vi "CAN.FG.vi"(7 "Action":T1, 8 "error in (no error)":errorcluster, 10 "Diagnostics Basic Configuration":T2={"Interface"="", "Baud Rate"=0, "Diagnostic Protocol"=enum."GMLAN", "Transport Protocol"=enum."ISO TP - Normal Mode", "Transmit ID"=0, "Receive ID"=0, "Transmit Extension"=0, "Receive Extension"=0, "Receive UUDT ID"=0, "Enable Stream"=TRUE, "VW TP Channel ID"=0, "Fill Frame"=TRUE, "Fill Byte"=255, "Termination"=FALSE, "LIN Cluster"="ADCS_LIN_database", "NAD"=1, "IO Mode"=0, "Max DLC"=8, "FD Baud Rate"=0, "Timeout"=1000, "FD ISO Mode"=0, "DoIP Address"="", "DoIP Source Address"=3584, "DoIP Dynamic Port"=TRUE, "DoIP Version"=2} {"DoIP Version" items=["2010"=1, "2012"=2]; "DoIP Source Address" format="%.0x"; "FD ISO Mode" items=["ISO", "Non ISO", "ISO Legacy"]; "IO Mode" items=["CAN 2.0", "CAN FD", "CAN FD+BRS"]; "Fill Byte" format="%.0x"; "VW TP Channel ID" format="%.0x"; "Receive UUDT ID" format="%.0x"; "Receive Extension" format="%.0x"; "Transmit Extension" format="%.0x"; "Receive ID" format="%.0x"; "Transmit ID" format="%.0x"}, 11 "Device Item Ref in":T6 format="%.0x") -> (0 "error out":errorcluster, 2 "Diagnostics Basic Configuration":T2={"Interface"="", "Baud Rate"=0, "Diagnostic Protocol"=enum."GMLAN", "Transport Protocol"=enum."ISO TP - Normal Mode", "Transmit ID"=0, "Receive ID"=0, "Transmit Extension"=0, "Receive Extension"=0, "Receive UUDT ID"=0, "Enable Stream"=TRUE, "VW TP Channel ID"=0, "Fill Frame"=FALSE, "Fill Byte"=255, "Termination"=FALSE, "LIN Cluster"="ADCS_LIN_database", "NAD"=1, "IO Mode"=0, "Max DLC"=8, "FD Baud Rate"=0, "Timeout"=0, "FD ISO Mode"=0, "DoIP Address"="", "DoIP Source Address"=3584, "DoIP Dynamic Port"=TRUE, "DoIP Version"=2} {"DoIP Version" items=["2010"=1, "2012"=2]; "DoIP Source Address" format="%.0x"; "FD ISO Mode" items=["ISO", "Non ISO", "ISO Legacy"]; "IO Mode" items=["CAN 2.0", "CAN FD", "CAN FD+BRS"]; "Fill Byte" format="%.0x"; "VW TP Channel ID" format="%.0x"; "Receive UUDT ID" format="%.0x"; "Receive Extension" format="%.0x"; "Transmit Extension" format="%.0x"; "Receive ID" format="%.0x"; "Transmit ID" format="%.0x"}, 3 "Device Item Ref out":T6=18446744073709551615 format="%.0x")   [LabVIEW 2019, in "Diagnostics Addon System Explorer.lvlib"]
uses:
  Diagnostics Addon System Explorer.lvlib
  <vilib>/NI VeriStand/Custom Device API/Custom Device Item Ref.ctl
  Addon Shared/Types/CAN.ctl
  Addon Shared/Types/CAN.Interface.ctl
  Addon Shared/Types/Protocol.ctl
  Addon Shared/Types/Transport.ctl
  Types/FG.Action.ctl
  Addon Shared/SubVIs/Constants.vi
  <vilib>/NI VeriStand/Custom Device API/Get Item Property (String).vi
  <vilib>/NI VeriStand/Custom Device API/Get Item Property (Variant).vi
  <vilib>/NI VeriStand/Custom Device API/Get Item Property (U32).vi
  <vilib>/NI VeriStand/Custom Device API/Get Item Property (Boolean).vi
  <vilib>/NI/NI VeriStand Advanced SysDef API/_SubVIs/SysDef.Property.Set.String.vi
  <vilib>/NI/NI VeriStand Advanced SysDef API/_SubVIs/SysDef.Property.Set.Variant.vi
  <vilib>/NI/NI VeriStand Advanced SysDef API/_SubVIs/SysDef.Property.Set.U32.vi
  <vilib>/NI/NI VeriStand Advanced SysDef API/_SubVIs/SysDef.Property.Set.Boolean.vi
  Addon Shared/Diagnostics Addon Shared.lvlib
  <vilib>/NI VeriStand/Custom Device API/Custom Device API.lvlib
  <vilib>/NI/NI VeriStand Advanced SysDef API/SysDef API/Advanced System Definition.lvlib
  <vilib>/NI/NI VeriStand Advanced SysDef API/_SubVIs/SysDef.Property.Set.U16.vi
  <vilib>/NI VeriStand/Custom Device API/Get Item Property (U16).vi
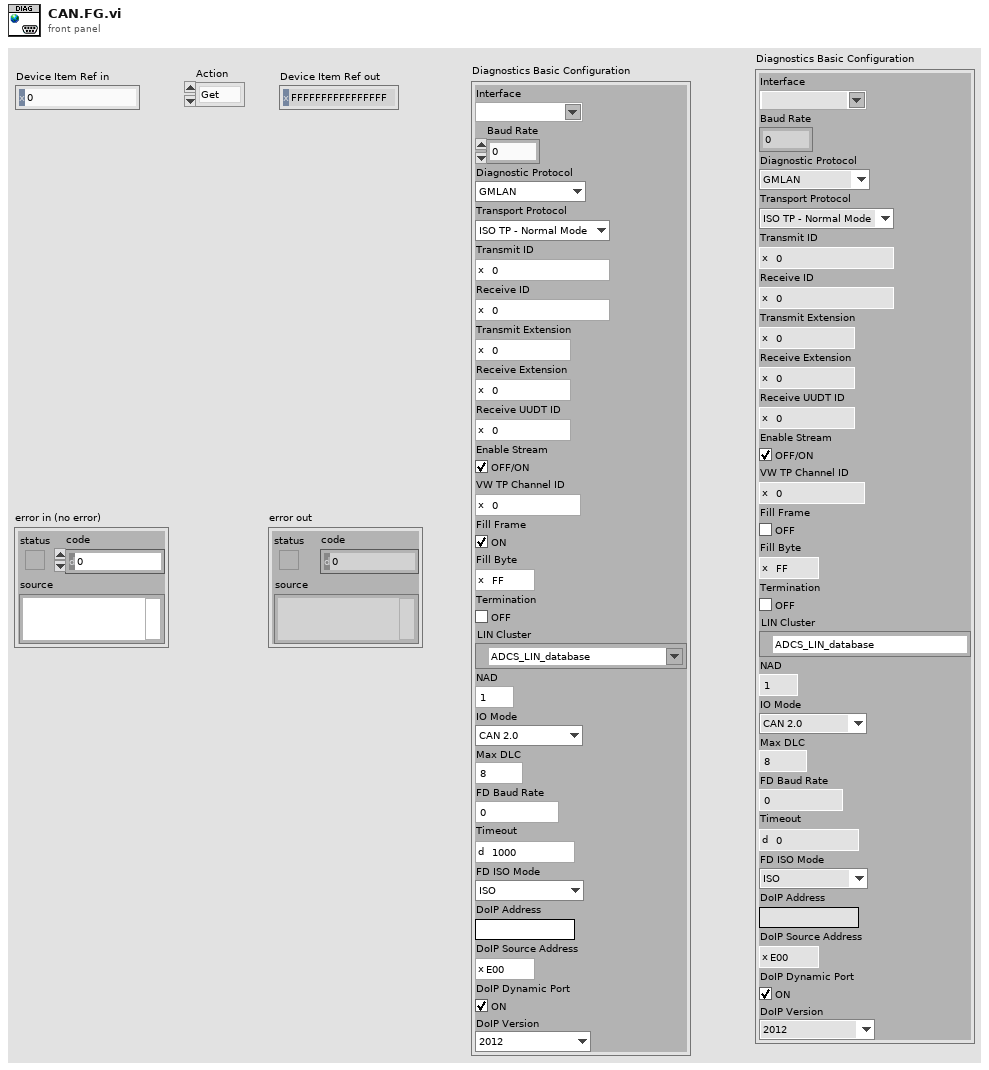
[diagram p1: front panel]
types:
  T1 = typedef "Diagnostics Addon System Explorer.lvlib/FG.Action.ctl" = enum16{"Get", "Set"}
  T2 = typedef "Diagnostics Addon Shared.lvlib/CAN.ctl" = cluster{"Interface":T3, "Baud Rate":u64, "Diagnostic Protocol":T4, "Transport Protocol":T5, "Transmit ID":u32, "Receive ID":u32, "Transmit Extension":u8, "Receive Extension":u8, "Receive UUDT ID":u32, "Enable Stream":bool, "VW TP Channel ID":u32, "Fill Frame":bool, "Fill Byte":u8, "Termination":bool, "LIN Cluster":refnum<k21>, "NAD":u8, "IO Mode":u32, "Max DLC":u16, "FD Baud Rate":u64, "Timeout":u32, "FD ISO Mode":u32, "DoIP Address":string, "DoIP Source Address":u16, "DoIP Dynamic Port":bool, "DoIP Version":u16}
  T3 = typedef "Diagnostics Addon Shared.lvlib/CAN.Interface.ctl" = string
  T4 = typedef "Diagnostics Addon Shared.lvlib/Protocol.ctl" = enum16{"GMLAN", "KWP-2000", "UDS", "User-Defined"}
  T5 = typedef "Diagnostics Addon Shared.lvlib/Transport.ctl" = enum16{"ISO TP - Normal Mode", "ISO TP - Mixed Mode", "VW TP 2.0", "Diagnostics on IP", "ISO TP LIN"}
  T6 = typedef "Custom Device API.lvlib/Custom Device Item Ref.ctl" = u64
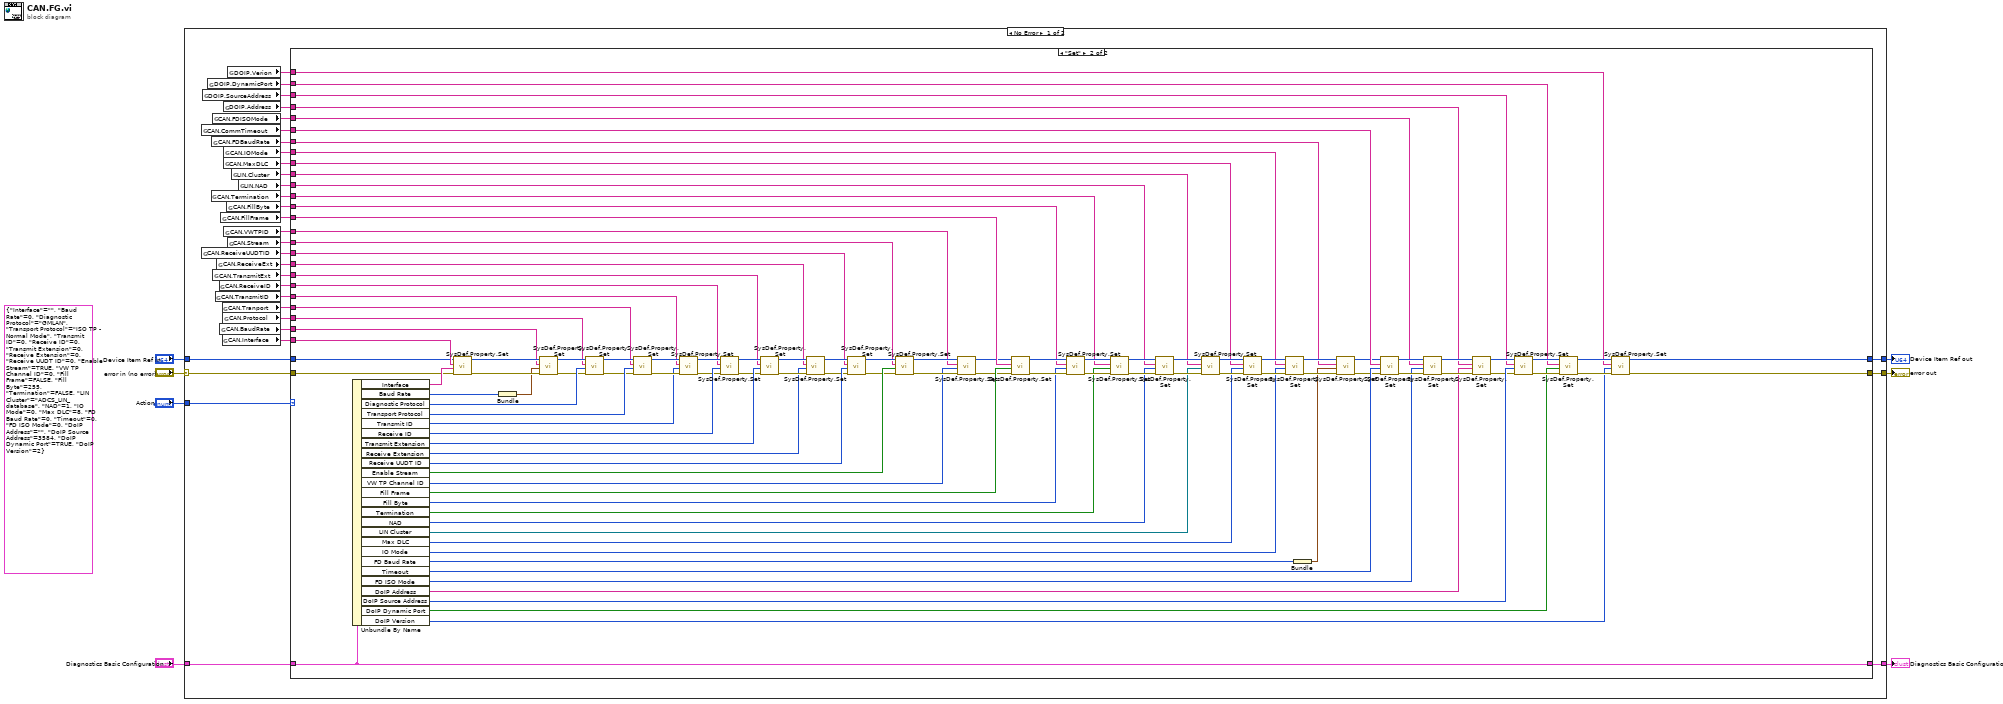
[diagram p0: block diagram]
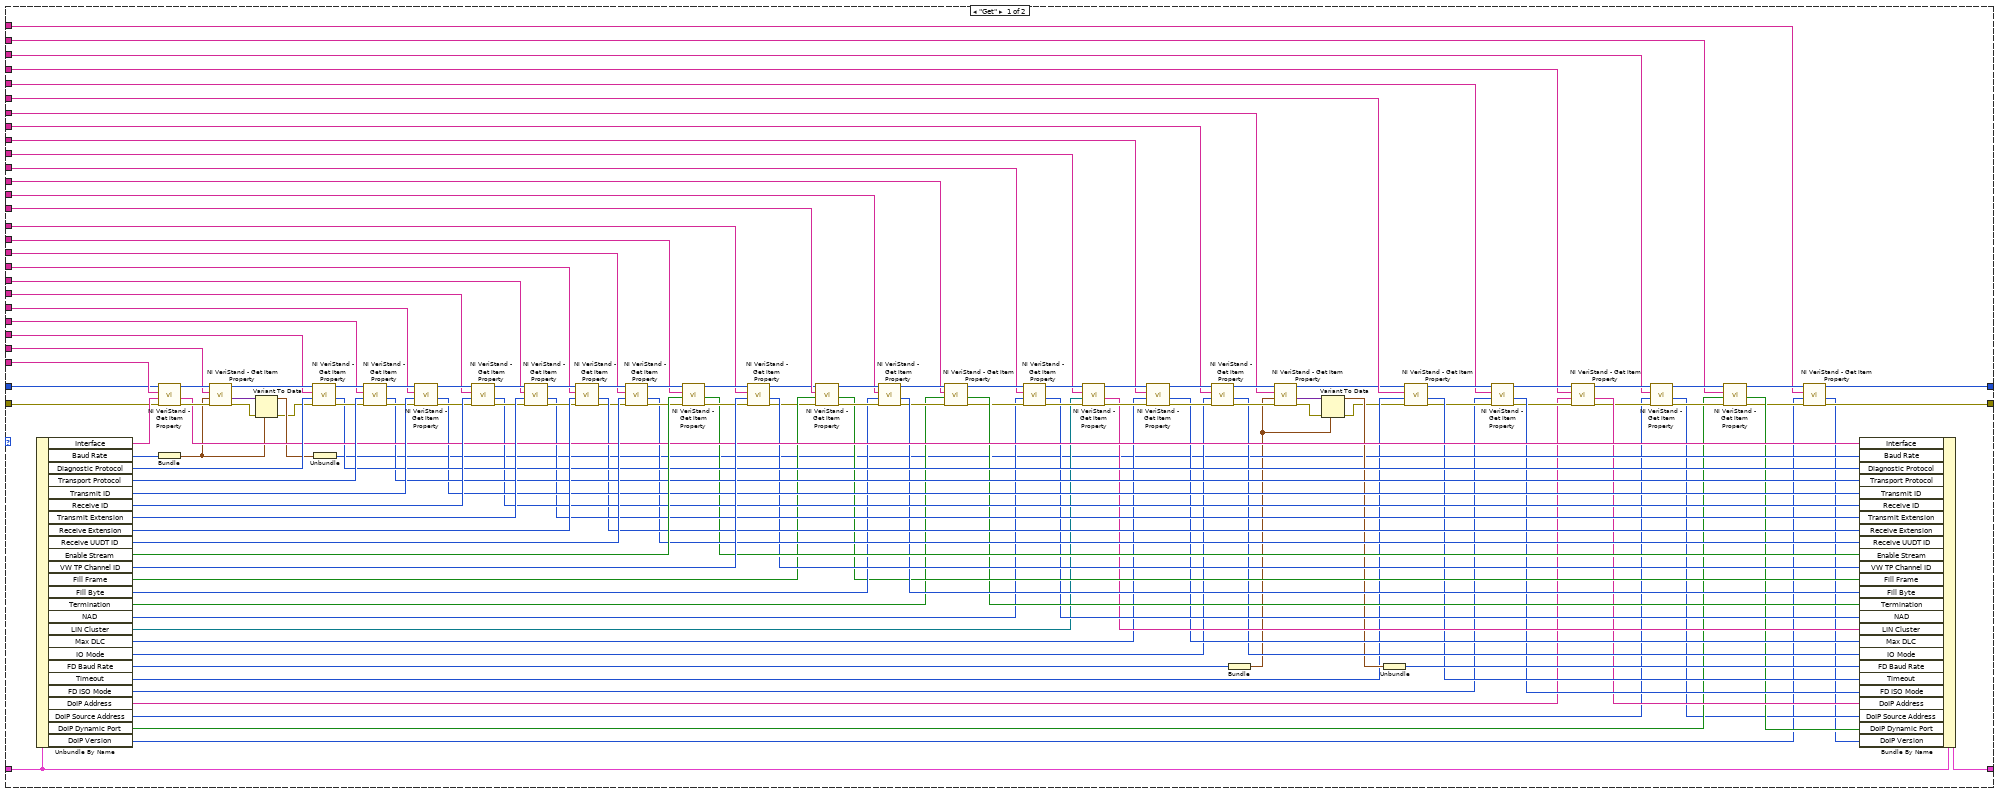
[diagram p2: hidden frame]
diagram:
  (unwired) T2 {"Interface"="", "Baud Rate"=0, "Diagnostic Protocol"=enum."GMLAN", "Transport Protocol"=enum."ISO TP - Normal Mode", "Transmit ID"=0, "Receive ID"=0, "Transmit Extension"=0, "Receive Extension"=0, "Receive UUDT ID"=0, "Enable Stream"=TRUE, "VW TP Channel ID"=0, "Fill Frame"=FALSE, "Fill Byte"=255, "Termination"=FALSE, "LIN Cluster"="ADCS_LIN_database", "NAD"=1, "IO Mode"=0, "Max DLC"=8, "FD Baud Rate"=0, "Timeout"=0, "FD ISO Mode"=0, "DoIP Address"="", "DoIP Source Address"=3584, "DoIP Dynamic Port"=TRUE, "DoIP Version"=2} ("Diagnostics Basic Configuraiton 2")
  n1 = case shown="No Error" "error in (no error)" {
    selector: "error in (no error)" -> [w39 w282]
    tunnel: "Device Item Ref in" -> [w38 w283]
    tunnel: [w37 w283] -> w4
    tunnel: [w36 w282] -> w5
    tunnel: [w35 _] -> w3
    tunnel: "Diagnostics Basic Configuration" -> [w34 _]
    tunnel: "Action" -> [w33 _]
    frame No Error {
      n2 = global read "Constants.vi" "CAN.CommTimeout"() -> (w13:string)
      n3 = global read "Constants.vi" "CAN.ReceiveUUDTID"() -> (w24:string)
      n4 = global read "Constants.vi" "DOIP.SourceAddress"() -> (w10:string)
      n5 = global read "Constants.vi" "DOIP.DynamicPort"() -> (w9:string)
      n6 = global read "Constants.vi" "CAN.Termination"() -> (w19:string)
      n7 = global read "Constants.vi" "CAN.FDBaudRate"() -> (w18:string)
      n8 = global read "Constants.vi" "CAN.FDISOMode"() -> (w12:string)
      n9 = global read "Constants.vi" "CAN.TransmitExt"() -> (w26:string)
      n10 = global read "Constants.vi" "CAN.TransmitID"() -> (w28:string)
      n11 = global read "Constants.vi" "CAN.ReceiveExt"() -> (w25:string)
      n12 = global read "Constants.vi" "CAN.ReceiveID"() -> (w27:string)
      n13 = global read "Constants.vi" "CAN.BaudRate"() -> (w31:string)
      n14 = global read "Constants.vi" "CAN.FillFrame"() -> (w21:string)
      n15 = global read "Constants.vi" "CAN.Tranport"() -> (w29:string)
      n16 = global read "Constants.vi" "CAN.Interface"() -> (w32:string)
      n17 = global read "Constants.vi" "CAN.Protocol"() -> (w30:string)
      n18 = global read "Constants.vi" "DOIP.Address"() -> (w11:string)
      n19 = global read "Constants.vi" "CAN.MaxDLC"() -> (w16:string)
      n20 = global read "Constants.vi" "CAN.IOMode"() -> (w17:string)
      n21 = global read "Constants.vi" "CAN.VWTPID"() -> (w22:string)
      n22 = global read "Constants.vi" "CAN.FillByte"() -> (w20:string)
      n23 = global read "Constants.vi" "CAN.Stream"() -> (w23:string)
      n24 = global read "Constants.vi" "DOIP.Verion"() -> (w8:string)
      n25 = global read "Constants.vi" "LIN.Cluster"() -> (w15:string)
      n26 = global read "Constants.vi" "LIN.NAD"() -> (w14:string)
      n27 = case shown="\"Set\"" w33 {
        tunnel: w39 -> [w110 w228]
        tunnel: w38 -> [w109 w227]
        tunnel: [w44 w179] -> w37
        tunnel: [w43 w181] -> w36
        tunnel: [w175 w281] -> w35
        tunnel: w34 -> [w176 w281]
        tunnel: w32 -> [w134 w249]
        tunnel: w31 -> [w133 w248]
        tunnel: w30 -> [w132 w247]
        tunnel: w29 -> [w131 w246]
        tunnel: w28 -> [w130 w245]
        tunnel: w27 -> [w129 w244]
        tunnel: w26 -> [w128 w243]
        tunnel: w25 -> [w127 w242]
        tunnel: w24 -> [w126 w241]
        tunnel: w23 -> [w125 w240]
        tunnel: w22 -> [w124 w239]
        tunnel: w21 -> [w117 w233]
        tunnel: w20 -> [w116 w234]
        tunnel: w19 -> [w111 w230]
        tunnel: w14 -> [w98 w211]
        tunnel: w15 -> [w97 w210]
        tunnel: w16 -> [w96 w209]
        tunnel: w17 -> [w95 w208]
        tunnel: w18 -> [w94 w207]
        tunnel: w13 -> [w71 w203]
        tunnel: w12 -> [w62 w196]
        tunnel: w11 -> [w57 w191]
        tunnel: w10 -> [w48 w184]
        tunnel: w9 -> [w47 w183]
        tunnel: w8 -> [w40 w177]
        frame "Get" {
          n28 = Unbundle By Name(w176) -> ("Interface"=w174:T3, "Baud Rate"=w173:u64, "Diagnostic Protocol"=w172:T4, "Transport Protocol"=w171:T5, "Transmit ID"=w170:u32, "Receive ID"=w169:u32, "Transmit Extension"=w168:u8, "Receive Extension"=w167:u8, "Receive UUDT ID"=w166:u32, "Enable Stream"=w165:bool, "VW TP Channel ID"=w164:u32, "Fill Frame"=w121:bool, "Fill Byte"=w120:u8, "Termination"=w113:bool, "NAD"=w93:u8, "LIN Cluster"=w91:refnum<k21>, "Max DLC"=w87:u16, "IO Mode"=w86:u32, "FD Baud Rate"=w85:u64, "Timeout"=w72:u32, "FD ISO Mode"=w64:u32, "DoIP Address"=w58:string, "DoIP Source Address"=w52:u16, "DoIP Dynamic Port"=w51:bool, "DoIP Version"=w41:u16)
          n29 = call-poly <vilib>:"NI VeriStand - Get Item Property.vi"("error in (no error)"=w110, "Default Value"=w174, "Property Name"=w134, "Item Ref in"=w109) -> ("error out"=w146:errorcluster, "Value"=w145:string, "Item Ref out"=w163:T6)  [unwired: 4 in, 1 out]
          n30 = Bundle("Baud Rate"=w173) -> (w76:cluster{"Baud Rate":u64})  [unwired: 1 in]
          n31 = call-poly <vilib>:"NI VeriStand - Get Item Property.vi"("error in (no error)"=w146, "Default Value"=w76, "Property Name"=w133, "Item Ref in"=w163) -> ("error out"=w79:errorcluster, "Value"=w81:variant, "Item Ref out"=w162:T6)  [unwired: 4 in, 1 out]
          n32 = Variant To Data(error in=w79, type=w76, Variant=w81) -> (data=w80:cluster{"Baud Rate":u64}, error out=w78:errorcluster)
          n33 = call-poly <vilib>:"NI VeriStand - Get Item Property.vi"("error in (no error)"=w78, "Default Value"=w172, "Property Name"=w132, "Item Ref in"=w162) -> ("error out"=w147:errorcluster, "Value"=w144:u32, "Item Ref out"=w161:T6)  [unwired: 4 in, 1 out]
          n34 = Unbundle(w80) -> ("Baud Rate"=w75:u64)
          n35 = call-poly <vilib>:"NI VeriStand - Get Item Property.vi"("error in (no error)"=w147, "Default Value"=w171, "Property Name"=w131, "Item Ref in"=w161) -> ("error out"=w148:errorcluster, "Value"=w143:u32, "Item Ref out"=w160:T6)  [unwired: 4 in, 1 out]
          n36 = call-poly <vilib>:"NI VeriStand - Get Item Property.vi"("error in (no error)"=w148, "Default Value"=w170, "Property Name"=w130, "Item Ref in"=w160) -> ("error out"=w149:errorcluster, "Value"=w142:u32, "Item Ref out"=w159:T6)  [unwired: 4 in, 1 out]
          n37 = call-poly <vilib>:"NI VeriStand - Get Item Property.vi"("error in (no error)"=w149, "Default Value"=w169, "Property Name"=w129, "Item Ref in"=w159) -> ("error out"=w150:errorcluster, "Value"=w141:u32, "Item Ref out"=w158:T6)  [unwired: 4 in, 1 out]
          n38 = call-poly <vilib>:"NI VeriStand - Get Item Property.vi"("error in (no error)"=w150, "Default Value"=w168, "Property Name"=w128, "Item Ref in"=w158) -> ("error out"=w151:errorcluster, "Value"=w140:u32, "Item Ref out"=w157:T6)  [unwired: 4 in, 1 out]
          n39 = call-poly <vilib>:"NI VeriStand - Get Item Property.vi"("error in (no error)"=w151, "Default Value"=w167, "Property Name"=w127, "Item Ref in"=w157) -> ("error out"=w138:errorcluster, "Value"=w139:u32, "Item Ref out"=w156:T6)  [unwired: 4 in, 1 out]
          n40 = call-poly <vilib>:"NI VeriStand - Get Item Property.vi"("error in (no error)"=w138, "Default Value"=w166, "Property Name"=w126, "Item Ref in"=w156) -> ("error out"=w152:errorcluster, "Value"=w137:u32, "Item Ref out"=w155:T6)  [unwired: 4 in, 1 out]
          n41 = call-poly <vilib>:"NI VeriStand - Get Item Property.vi"("error in (no error)"=w152, "Default Value"=w165, "Property Name"=w125, "Item Ref in"=w155) -> ("error out"=w153:errorcluster, "Value"=w136:bool, "Item Ref out"=w154:T6)  [unwired: 4 in, 1 out]
          n42 = call-poly <vilib>:"NI VeriStand - Get Item Property.vi"("error in (no error)"=w153, "Default Value"=w164, "Property Name"=w124, "Item Ref in"=w154) -> ("error out"=w69:errorcluster, "Value"=w135:u32, "Item Ref out"=w70:T6)  [unwired: 4 in, 1 out]
          n43 = call-poly <vilib>:"NI VeriStand - Get Item Property.vi"("error in (no error)"=w69, "Default Value"=w121, "Property Name"=w117, "Item Ref in"=w70) -> ("error out"=w123:errorcluster, "Value"=w118:bool, "Item Ref out"=w122:T6)  [unwired: 4 in, 1 out]
          n44 = call-poly <vilib>:"NI VeriStand - Get Item Property.vi"("error in (no error)"=w123, "Default Value"=w120, "Property Name"=w116, "Item Ref in"=w122) -> ("error out"=w114:errorcluster, "Value"=w119:u32, "Item Ref out"=w115:T6)  [unwired: 4 in, 1 out]
          n45 = call-poly <vilib>:"NI VeriStand - Get Item Property.vi"("error in (no error)"=w114, "Default Value"=w113, "Property Name"=w111, "Item Ref in"=w115) -> ("error out"=w104:errorcluster, "Value"=w112:bool, "Item Ref out"=w102:T6)  [unwired: 4 in, 1 out]
          n46 = call-poly <vilib>:"NI VeriStand - Get Item Property.vi"("error in (no error)"=w104, "Default Value"=w93, "Property Name"=w98, "Item Ref in"=w102) -> ("error out"=w108:errorcluster, "Value"=w92:u32, "Item Ref out"=w101:T6)  [unwired: 4 in, 1 out]
          n47 = call-poly <vilib>:"NI VeriStand - Get Item Property.vi"("error in (no error)"=w108, "Default Value"=w91, "Property Name"=w97, "Item Ref in"=w101) -> ("error out"=w107:errorcluster, "Value"=w90:string, "Item Ref out"=w100:T6)  [unwired: 4 in, 1 out]
          n48 = call-poly <vilib>:"NI VeriStand - Get Item Property.vi"("error in (no error)"=w107, "Default Value"=w87, "Property Name"=w96, "Item Ref in"=w100) -> ("error out"=w106:errorcluster, "Value"=w89:u32, "Item Ref out"=w99:T6)  [unwired: 4 in, 1 out]
          n49 = call-poly <vilib>:"NI VeriStand - Get Item Property.vi"("error in (no error)"=w106, "Default Value"=w86, "Property Name"=w95, "Item Ref in"=w99) -> ("error out"=w105:errorcluster, "Value"=w88:u32, "Item Ref out"=w103:T6)  [unwired: 4 in, 1 out]
          n50 = Bundle("FD Baud Rate"=w85) -> (w74:cluster{"FD Baud Rate":u64})  [unwired: 1 in]
          n51 = call-poly <vilib>:"NI VeriStand - Get Item Property.vi"("error in (no error)"=w105, "Default Value"=w74, "Property Name"=w94, "Item Ref in"=w103) -> ("error out"=w83:errorcluster, "Value"=w84:variant, "Item Ref out"=w68:T6)  [unwired: 4 in, 1 out]
          n52 = Variant To Data(error in=w83, type=w74, Variant=w84) -> (data=w82:cluster{"FD Baud Rate":u64}, error out=w67:errorcluster)
          n53 = Unbundle(w82) -> ("FD Baud Rate"=w77:u64)
          n54 = call-poly <vilib>:"NI VeriStand - Get Item Property.vi"("error in (no error)"=w67, "Default Value"=w72, "Property Name"=w71, "Item Ref in"=w68) -> ("error out"=w66:errorcluster, "Value"=w73:u32, "Item Ref out"=w65:T6)  [unwired: 4 in, 1 out]
          n55 = call-poly <vilib>:"NI VeriStand - Get Item Property.vi"("error in (no error)"=w66, "Default Value"=w64, "Property Name"=w62, "Item Ref in"=w65) -> ("error out"=w61:errorcluster, "Value"=w63:u32, "Item Ref out"=w60:T6)  [unwired: 4 in, 1 out]
          n56 = call-poly <vilib>:"NI VeriStand - Get Item Property.vi"("error in (no error)"=w61, "Default Value"=w58, "Property Name"=w57, "Item Ref in"=w60) -> ("error out"=w56:errorcluster, "Value"=w59:string, "Item Ref out"=w55:T6)  [unwired: 4 in, 1 out]
          n57 = call-poly <vilib>:"NI VeriStand - Get Item Property.vi"("error in (no error)"=w56, "Default Value"=w52, "Property Name"=w48, "Item Ref in"=w55) -> ("error out"=w53:errorcluster, "Value"=w49:u16, "Item Ref out"=w54:T6)  [unwired: 4 in, 1 out]
          n58 = call-poly <vilib>:"NI VeriStand - Get Item Property.vi"("error in (no error)"=w53, "Default Value"=w51, "Property Name"=w47, "Item Ref in"=w54) -> ("error out"=w46:errorcluster, "Value"=w50:bool, "Item Ref out"=w45:T6)  [unwired: 4 in, 1 out]
          n59 = call-poly <vilib>:"NI VeriStand - Get Item Property.vi"("error in (no error)"=w46, "Default Value"=w41, "Property Name"=w40, "Item Ref in"=w45) -> ("error out"=w43:errorcluster, "Value"=w42:u32, "Item Ref out"=w44:T6)  [unwired: 4 in, 1 out]
          n60 = Bundle By Name(cluster=w176, "Interface"=w145, "Baud Rate"=w75, "Diagnostic Protocol"=w144, "Transport Protocol"=w143, "Transmit ID"=w142, "Receive ID"=w141, "Transmit Extension"=w140, "Receive Extension"=w139, "Receive UUDT ID"=w137, "Enable Stream"=w136, "VW TP Channel ID"=w135, "Fill Frame"=w118, "Fill Byte"=w119, "Termination"=w112, "NAD"=w92, "LIN Cluster"=w90, "Max DLC"=w89, "IO Mode"=w88, "FD Baud Rate"=w77, "Timeout"=w73, "FD ISO Mode"=w63, "DoIP Address"=w59, "DoIP Source Address"=w49, "DoIP Dynamic Port"=w50, "DoIP Version"=w42) -> (w175:T2)
        }
        frame "Set" {
          n61 = Unbundle By Name(w281) -> ("Interface"=w280:T3, "Baud Rate"=w277:u64, "Diagnostic Protocol"=w270:T4, "Transport Protocol"=w269:T5, "Transmit ID"=w268:u32, "Receive ID"=w267:u32, "Transmit Extension"=w266:u8, "Receive Extension"=w265:u8, "Receive UUDT ID"=w264:u32, "Enable Stream"=w263:bool, "VW TP Channel ID"=w262:u32, "Fill Frame"=w236:bool, "Fill Byte"=w235:u8, "Termination"=w229:bool, "NAD"=w216:u8, "LIN Cluster"=w215:refnum<k21>, "Max DLC"=w214:u16, "IO Mode"=w213:u32, "FD Baud Rate"=w212:u64, "Timeout"=w204:u32, "FD ISO Mode"=w195:u32, "DoIP Address"=w192:string, "DoIP Source Address"=w190:u16, "DoIP Dynamic Port"=w185:bool, "DoIP Version"=w178:u16)
          n62 = call-poly <vilib>:"SysDef.Property.Set.vi"("error in (no error)"=w228, "Value"=w280, "Property Name"=w249, "nodeID"=w227) -> ("error out"=w278:errorcluster, "nodeID out"=w279:u64)  [unwired: 6 in]
          n63 = Bundle("Baud Rate"=w277) -> (w205:cluster{"Baud Rate":u64})  [unwired: 1 in]
          n64 = call-poly <vilib>:"SysDef.Property.Set.vi"("error in (no error)"=w278, "Value"=w205, "Property Name"=w248, "nodeID"=w279) -> ("error out"=w250:errorcluster, "nodeID out"=w261:u64)  [unwired: 6 in]
          n65 = call-poly <vilib>:"SysDef.Property.Set.vi"("error in (no error)"=w250, "Value"=w270, "Property Name"=w247, "nodeID"=w261) -> ("error out"=w251:errorcluster, "nodeID out"=w260:u64)  [unwired: 6 in]
          n66 = call-poly <vilib>:"SysDef.Property.Set.vi"("error in (no error)"=w251, "Value"=w269, "Property Name"=w246, "nodeID"=w260) -> ("error out"=w276:errorcluster, "nodeID out"=w275:u64)  [unwired: 6 in]
          n67 = call-poly <vilib>:"SysDef.Property.Set.vi"("error in (no error)"=w276, "Value"=w268, "Property Name"=w245, "nodeID"=w275) -> ("error out"=w252:errorcluster, "nodeID out"=w259:u64)  [unwired: 6 in]
          n68 = call-poly <vilib>:"SysDef.Property.Set.vi"("error in (no error)"=w252, "Value"=w267, "Property Name"=w244, "nodeID"=w259) -> ("error out"=w253:errorcluster, "nodeID out"=w258:u64)  [unwired: 6 in]
          n69 = call-poly <vilib>:"SysDef.Property.Set.vi"("error in (no error)"=w253, "Value"=w266, "Property Name"=w243, "nodeID"=w258) -> ("error out"=w272:errorcluster, "nodeID out"=w271:u64)  [unwired: 6 in]
          n70 = call-poly <vilib>:"SysDef.Property.Set.vi"("error in (no error)"=w272, "Value"=w265, "Property Name"=w242, "nodeID"=w271) -> ("error out"=w254:errorcluster, "nodeID out"=w257:u64)  [unwired: 6 in]
          n71 = call-poly <vilib>:"SysDef.Property.Set.vi"("error in (no error)"=w254, "Value"=w264, "Property Name"=w241, "nodeID"=w257) -> ("error out"=w255:errorcluster, "nodeID out"=w256:u64)  [unwired: 6 in]
          n72 = call-poly <vilib>:"SysDef.Property.Set.vi"("error in (no error)"=w255, "Value"=w263, "Property Name"=w240, "nodeID"=w256) -> ("error out"=w273:errorcluster, "nodeID out"=w274:u64)  [unwired: 6 in]
          n73 = call-poly <vilib>:"SysDef.Property.Set.vi"("error in (no error)"=w273, "Value"=w262, "Property Name"=w239, "nodeID"=w274) -> ("error out"=w202:errorcluster, "nodeID out"=w201:u64)  [unwired: 6 in]
          n74 = call-poly <vilib>:"SysDef.Property.Set.vi"("error in (no error)"=w202, "Value"=w236, "Property Name"=w233, "nodeID"=w201) -> ("error out"=w238:errorcluster, "nodeID out"=w237:u64)  [unwired: 6 in]
          n75 = call-poly <vilib>:"SysDef.Property.Set.vi"("error in (no error)"=w238, "Value"=w235, "Property Name"=w234, "nodeID"=w237) -> ("error out"=w232:errorcluster, "nodeID out"=w231:u64)  [unwired: 6 in]
          n76 = call-poly <vilib>:"SysDef.Property.Set.vi"("error in (no error)"=w232, "Value"=w229, "Property Name"=w230, "nodeID"=w231) -> ("error out"=w226:errorcluster, "nodeID out"=w225:u64)  [unwired: 6 in]
          n77 = call-poly <vilib>:"SysDef.Property.Set.vi"("error in (no error)"=w226, "Value"=w216, "Property Name"=w211, "nodeID"=w225) -> ("error out"=w224:errorcluster, "nodeID out"=w223:u64)  [unwired: 6 in]
          n78 = call-poly <vilib>:"SysDef.Property.Set.vi"("error in (no error)"=w224, "Value"=w215, "Property Name"=w210, "nodeID"=w223) -> ("error out"=w221:errorcluster, "nodeID out"=w222:u64)  [unwired: 6 in]
          n79 = call-poly <vilib>:"SysDef.Property.Set.vi"("error in (no error)"=w221, "Value"=w214, "Property Name"=w209, "nodeID"=w222) -> ("error out"=w217:errorcluster, "nodeID out"=w220:u64)  [unwired: 6 in]
          n80 = call-poly <vilib>:"SysDef.Property.Set.vi"("error in (no error)"=w217, "Value"=w213, "Property Name"=w208, "nodeID"=w220) -> ("error out"=w218:errorcluster, "nodeID out"=w219:u64)  [unwired: 6 in]
          n81 = Bundle("FD Baud Rate"=w212) -> (w206:cluster{"FD Baud Rate":u64})  [unwired: 1 in]
          n82 = call-poly <vilib>:"SysDef.Property.Set.vi"("error in (no error)"=w218, "Value"=w206, "Property Name"=w207, "nodeID"=w219) -> ("error out"=w200:errorcluster, "nodeID out"=w199:u64)  [unwired: 6 in]
          n83 = call-poly <vilib>:"SysDef.Property.Set.vi"("error in (no error)"=w200, "Value"=w204, "Property Name"=w203, "nodeID"=w199) -> ("error out"=w198:errorcluster, "nodeID out"=w197:u64)  [unwired: 6 in]
          n84 = call-poly <vilib>:"SysDef.Property.Set.vi"("error in (no error)"=w198, "Value"=w195, "Property Name"=w196, "nodeID"=w197) -> ("error out"=w194:errorcluster, "nodeID out"=w193:u64)  [unwired: 6 in]
          n85 = call-poly <vilib>:"SysDef.Property.Set.vi"("error in (no error)"=w194, "Value"=w192, "Property Name"=w191, "nodeID"=w193) -> ("error out"=w188:errorcluster, "nodeID out"=w189:u64)  [unwired: 6 in]
          n86 = call-poly <vilib>:"SysDef.Property.Set.vi"("error in (no error)"=w188, "Value"=w190, "Property Name"=w184, "nodeID"=w189) -> ("error out"=w187:errorcluster, "nodeID out"=w186:u64)  [unwired: 6 in]
          n87 = call-poly <vilib>:"SysDef.Property.Set.vi"("error in (no error)"=w187, "Value"=w185, "Property Name"=w183, "nodeID"=w186) -> ("error out"=w182:errorcluster, "nodeID out"=w180:u64)  [unwired: 6 in]
          n88 = call-poly <vilib>:"SysDef.Property.Set.vi"("error in (no error)"=w182, "Value"=w178, "Property Name"=w177, "nodeID"=w180) -> ("error out"=w181:errorcluster, "nodeID out"=w179:u64)  [unwired: 6 in]
        }
      }
    }
    frame Error {
    }
  }
  "error out" <- w5
  "Device Item Ref out" <- w4
  "Diagnostics Basic Configuration" <- w3
